vi "Show scan pass or fail.vi"(6 "Next Tray Cnt":u32, 8 "error in (no error)":errorcluster, 9 "Trays":u32, 10 "Tray number":u32, 11 "Passed?":bool) -> (0 "error out":errorcluster)   [LabVIEW 2013]
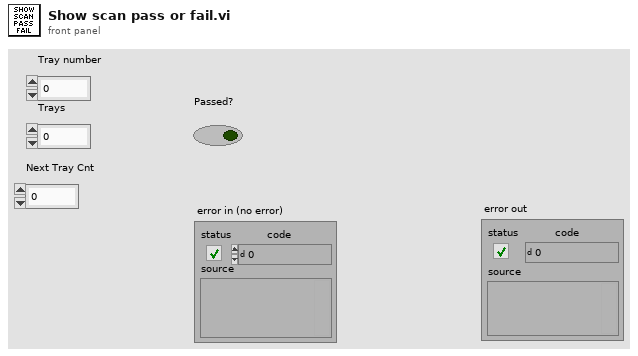
[diagram p1: front panel]
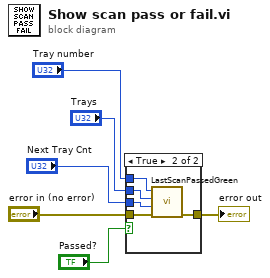
[diagram p0: block diagram]
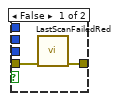
[diagram p2: hidden frame]
diagram:
  n1 = case shown="True" "Passed?" {
    tunnel: "error in (no error)" -> [w8 w13]
    tunnel: [w7 w12] -> w4
    tunnel: "Tray number" -> [_ w11]
    tunnel: "Trays" -> [_ w10]
    tunnel: "Next Tray Cnt" -> [_ w9]
    frame False {
      n2 = call "LastScanFailedRed.vi"("error in (no error)"=w8) -> ("error out"=w7:errorcluster)  [unwired: 10 in]
    }
    frame True {
      n3 = call "LastScanPassedGreen.vi"("error in (no error)"=w13, "Next Tray Cnt"=w9, "Trays"=w10, "Tray"=w11) -> ("error out"=w12:errorcluster)  [unwired: 7 in]
    }
  }
  "error out" <- w4
